vi "机械手.vi"() -> ()   [LabVIEW 2014]
uses:
  <vilib>/Utility/sysdir.llb/System Directory Type.ctl
  <vilib>/Instr/_visa.llb/VISA Configure Serial Port (Instr).vi
panel:
  in  "选项卡控件":enum32{" 肌电传感器电极", " 电机反馈", "FSR&弯曲传感器", "手动写入"}(tab)
  out "手势类型":dbl
  out "蓝牙状态":bool
  in  "接收串口":refnum<visa-resource-name>
  in  "?":bool
  out "肌电传感器电极":dbl(graph)
  out "肌电传感器电极 2":dbl(graph)
  out "肌电传感器电极 3":dbl(graph)
  out "肌电传感器电极 4":dbl(graph)
  out "肌电传感器电极 5":dbl(graph)
  out "肌电传感器电极 6":dbl(graph)
  out "肌电传感器电极 7":dbl(graph)
  out "肌电传感器电极 8":dbl(graph)
  in  "?":bool
  out "小指摆动电机电流":dbl
  out "无名指摆动电机电流":dbl
  out "中指摆动电机电流":dbl
  out "食指摆动电机电流":dbl
  out "拇指摆动电机电流":dbl
  out "拇指张合电机电流":dbl
  out "中指摆动电机转速":dbl(graph)
  out "无名指摆动电机转速":dbl(graph)
  out "小指摆动电机转速":dbl(graph)
  out "拇指张合电机转速":dbl(graph)
  out "拇指摆动电机转速":dbl(graph)
  out "食指摆动电机转速":dbl(graph)
  in  "?":bool
  out "复合":dynamicdata(graph)
  out "FSR4法向压力 4":dbl(graph)
  out "拇指弯曲度":dbl(graph)
  out "食指弯曲度":dbl(graph)
  out "中指弯曲度":dbl(graph)
  out "FSR1法向压力":dbl(graph)
  out "FSR2法向压力":dbl(graph)
  out "FSR3法向压力":dbl(graph)
  out "数值显示控件 6":dbl
  out "数值显示控件 5":dbl
  out "数值显示控件 4":dbl
  out "数值显示控件 3":dbl
  out "数值显示控件 2":dbl
  out "数值显示控件":dbl
  in  "?":bool
  in  "?":bool
  in  "?":bool
  in  "?":bool
  in  "?":bool
  in  "?":bool
  in  "?":bool
  in  "?":bool
  in  "小指摆动电机目标转速":dbl(knob) scale=-29.286..29.286 scale format="%#_4g"
  in  "无名指摆动电机目标转速":dbl(knob) scale=-29.286..29.286 scale format="%#_4g"
  in  "中指摆动电机目标转速":dbl(knob) scale=-29.286..29.286 scale format="%#_4g"
  in  "食指摆动电机目标转速":dbl(knob) scale=-29.286..29.286 scale format="%#_4g"
  in  "拇指摆动电机目标转速":dbl(knob) scale=-29.286..29.286 scale format="%#_4g"
  in  "拇指张合电机目标转速":dbl(knob) scale=-29.286..29.286 scale format="%#_4g"
  # "中南大学机电工程学院 复杂装备智能控制实验室  假肢手控制系统V2.0"
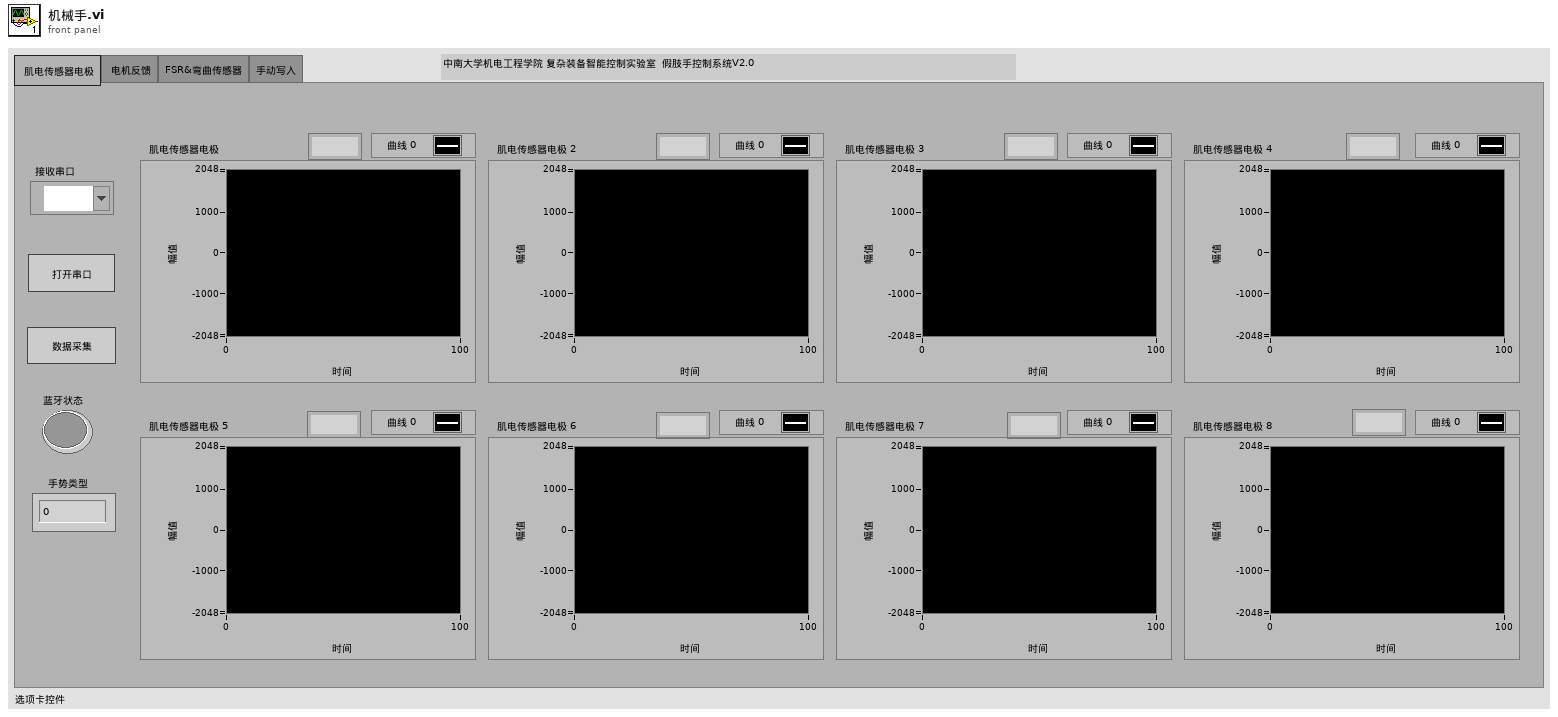
[diagram p1: front panel]
types:
  T1 = enum16{"open", "replace", "create", "open or create", "replace or create", "replace or create with confirmation"}
  T2 = typedef "System Directory Type.ctl" = i32
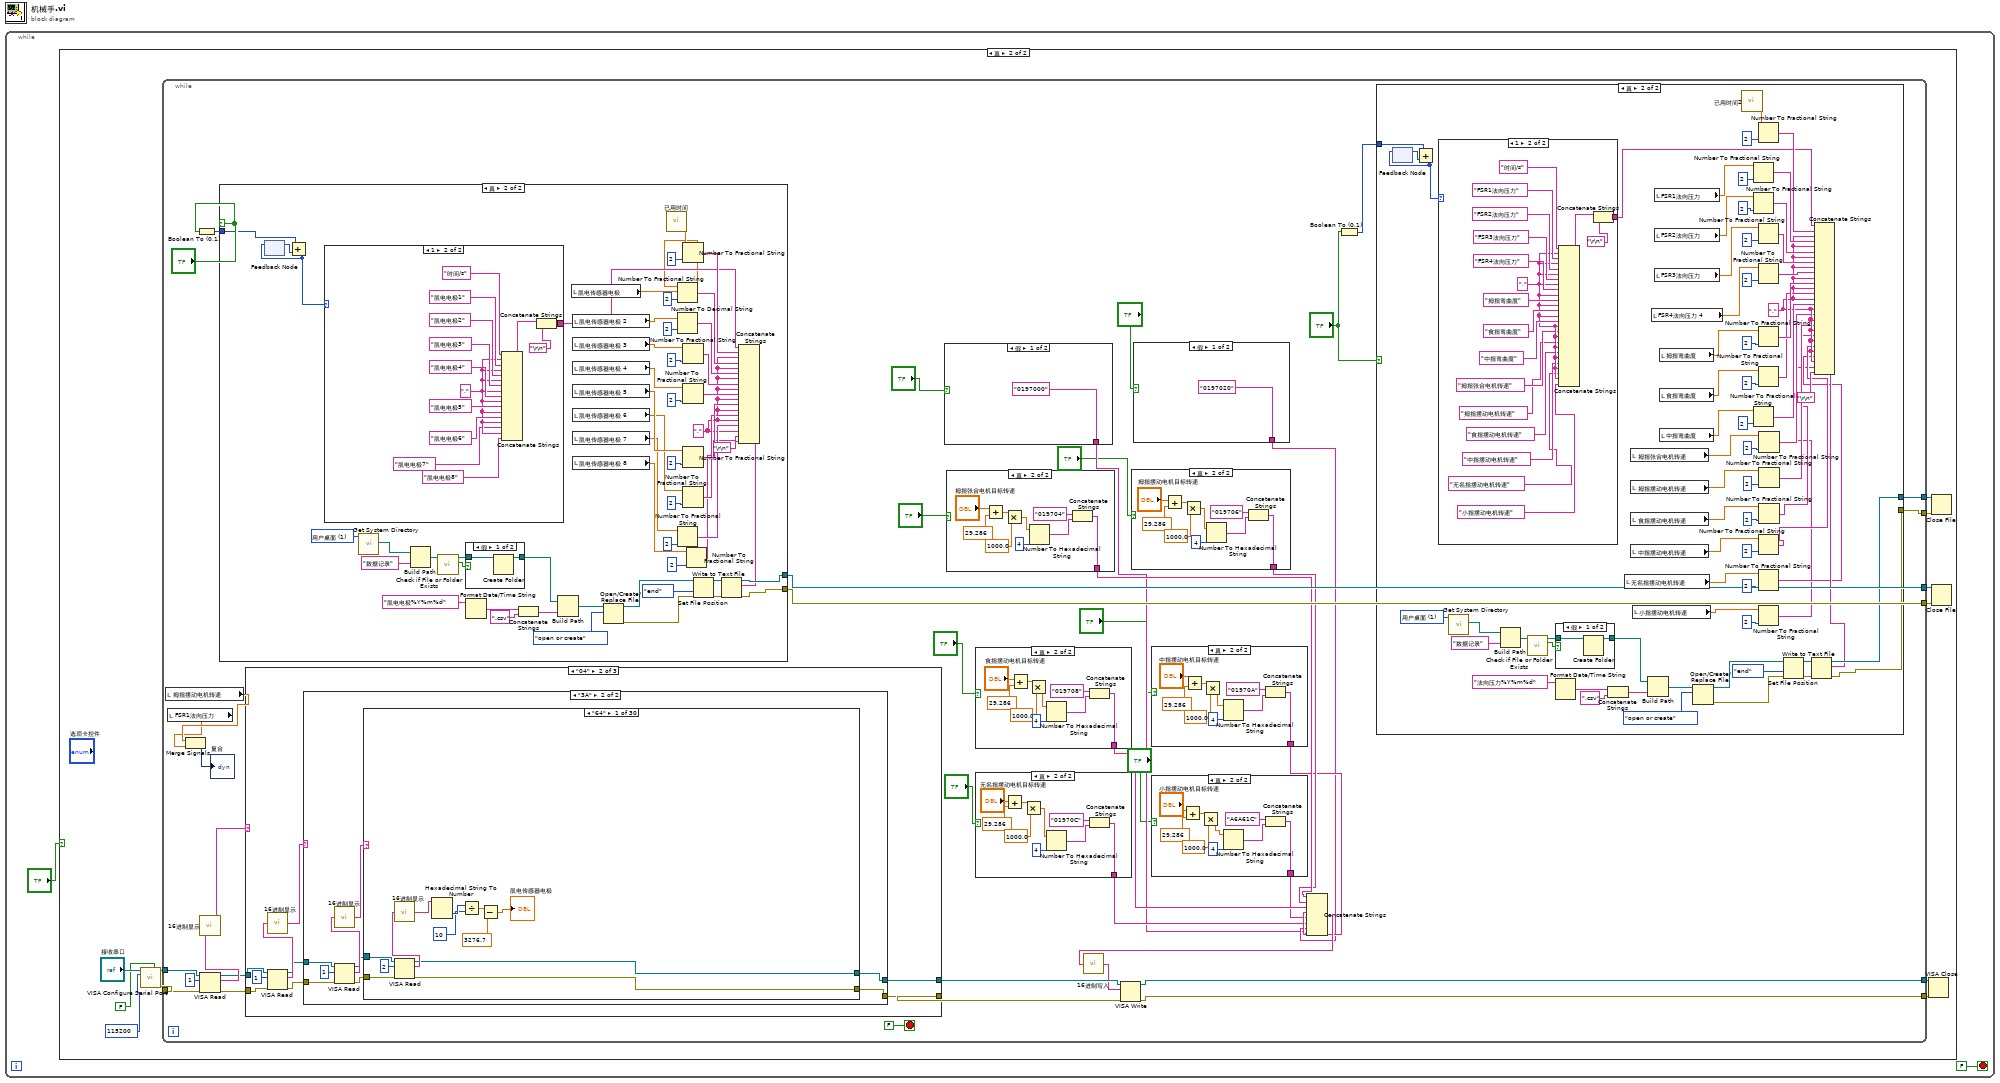
[diagram p0: block diagram]
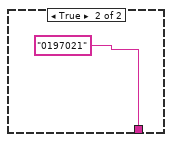
[diagram p6: hidden frame]
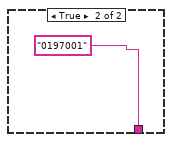
[diagram p7: hidden frame]
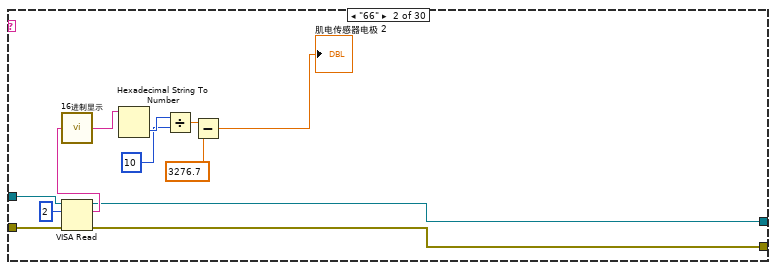
[diagram p19: hidden frame]
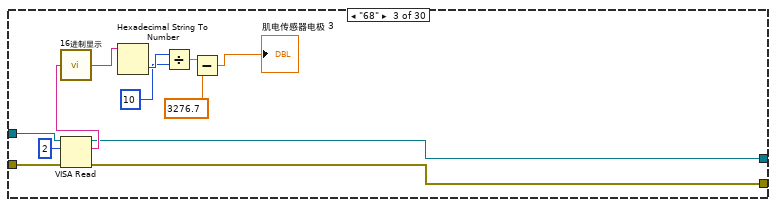
[diagram p20: hidden frame]
diagram:
  n1 = while {
    stop <- FALSE stop-if-true
    n2 = case shown="真" "?" {
      frame False {
      }
      frame True {
        n3 = call-poly "VISA Configure Serial Port"("VISA resource name"="接收串口", "Enable Termination\nChar (T)"=FALSE ("Enable Termination\nChar (T)"), "baud rate (9600)"=u32 115200) -> ("VISA resource name out"=w10:refnum<visa-resource-name>, "error out"=w9:errorcluster)  [unwired: 11 in]
        n4 = while {
          tunnel: w10 -> [w52]
          tunnel: w9 -> [w51]
          tunnel: [w37] -> w8
          tunnel: [w36] -> w7
          tunnel: [w44] -> w6
          tunnel: [w43] -> w5
          tunnel: [w17] -> w4
          tunnel: [w16] -> w3
          stop <- FALSE stop-if-true
          n5 = local read "拇指摆动电机转速"() -> (w41:dbl)
          n6 = local read "FSR1法向压力"() -> (w40:dbl)
          n7 = Merge Signals(w41, w40) -> (→"复合":dynamicdata)
          n8 = Boolean To (0,1)(Boolean="?") -> (0, 1=w46:i16)
          n9 = VISA Read(VISA resource name=w52, byte count=u32 1 ("字节总数"), error in (no error)=w51) -> (VISA resource name out=w48:refnum<visa-resource-name>, read buffer=w50:string, error out=w47:errorcluster)  [unwired: 1 out]
          n10 = call "16进制显示.vi"("输入"=w50) -> ("输出"=w49:string)
          n11 = case shown="真" "?" {
            tunnel: [_ w256] -> w44
            tunnel: [_ w255] -> w43
            tunnel: w46 -> [_ w254]
            frame False {
            }
            frame True {
              w203 = "," ("字符串")
              w231 = T2 1 items=["用户目录"=0, "用户桌面"=1, "用户文档"=2, "用户应用程序数据"=3, "用户设置"=4, "用户临时目录"=5, "公共文档"=6, "公共应用程序数据"=7, "公共设置"=8, "公共缓存"=13, "系统核心库"=9, "系统安装库"=10, "应用程序文件"=11, "启动盘根目录"=12] ("system directory type")
              n12 = feedback #1() -> (w233:i16)  [unwired: 1 in]
              n13 = Add(x=w254, y=w233) -> (x+y=w232:i16)
              n14 = feedback-in #1(w232) -> ()
              n15 = case shown="1" w232 {
                tunnel: [_ w261] -> w219
                frame 0, Default {
                }
                frame 1 {
                  w262 = "," ("字符串")
                  n16 = Concatenate Strings("时间/s" ("字符串"), w262, "肌电电极1" ("字符串"), w262, "肌电电极2" ("字符串"), w262, "肌电电极3" ("字符串"), w262, "肌电电极4" ("字符串"), w262, "肌电电极5" ("字符串"), w262, "肌电电极6" ("字符串"), w262, "肌电电极7" ("字符串"), w262, "肌电电极8" ("字符串")) -> (w260:string)
                  n17 = Concatenate Strings(w260, "\r\n") -> (w261:string)
                }
              }
              n18 = call <vilib>:"Get System Directory.vi"("system directory type"=w231) -> ("system directory"=w230:path)  [unwired: 10 in]
              n19 = Build Path(base path=w230, name or relative path="数据记录" ("名称或相对路径")) -> (appended path=w253:path)
              n20 = call <vilib>:"Check if File or Folder Exists.vi"("path"=w253) -> ("file or folder exists?"=w251:bool, "dup path"=w252:path)  [unwired: 8 in, 1 out]
              n21 = case shown="假" w251 {
                tunnel: w252 -> [w271 w272]
                tunnel: [w270 w272] -> w240
                frame False {
                  n22 = Create Folder(path (use dialog)=w271) -> (created path=w270:path)  [unwired: 2 in, 2 out]
                }
                frame True {
                }
              }
              n23 = Format Date/Time String(time format string (%c)="肌电电极%Y%m%d" ("时间格式字符串(%c)")) -> (date/time string=w239:string)  [unwired: 2 in]
              n24 = Concatenate Strings(w239, ".csv" ("字符串")) -> (w245:string)
              n25 = Build Path(base path=w240, name or relative path=w245) -> (appended path=w247:path)
              n26 = local read "肌电传感器电极"() -> (w217:dbl)
              n27 = local read "肌电传感器电极 2"() -> (w214:dbl)
              n28 = local read "肌电传感器电极 3"() -> (w213:dbl)
              n29 = local read "肌电传感器电极 4"() -> (w212:dbl)
              n30 = local read "肌电传感器电极 5"() -> (w211:dbl)
              n31 = local read "肌电传感器电极 6"() -> (w210:dbl)
              n32 = local read "肌电传感器电极 7"() -> (w209:dbl)
              n33 = local read "肌电传感器电极 8"() -> (w205:dbl)
              n34 = Open/Create/Replace File(file path (use dialog)=w247, operation (0:open)=T1."open or create" ("操作(0:open)")) -> (refnum out=w248:refnum<file>, error out=w249:errorcluster)  [unwired: 4 in, 1 out]
              n35 = call "已用时间"() -> ("Elapsed Time (s)"=w236:dbl)  [unwired: 12 in, 7 out]
              n36 = Number To Fractional String(number=w217, precision (6)=i16 2 ("精度(6)")) -> (F-format string=w221:string)  [unwired: 2 in]
              n37 = Number To Decimal String(number=w214, width (-)=i16 2 ("宽度(-)")) -> (decimal integer string=w208:string)
              n38 = Number To Fractional String(number=w209, precision (6)=i16 2 ("精度(6)")) -> (F-format string=w220:string)  [unwired: 2 in]
              n39 = Number To Fractional String(number=w236, precision (6)=i16 2 ("精度(6)")) -> (F-format string=w235:string)  [unwired: 2 in]
              n40 = Number To Fractional String(number=w213, precision (6)=i16 2 ("精度(6)")) -> (F-format string=w229:string)  [unwired: 2 in]
              n41 = Number To Fractional String(number=w212, precision (6)=i16 2 ("精度(6)")) -> (F-format string=w228:string)  [unwired: 2 in]
              n42 = Number To Fractional String(number=w211, precision (6)=i16 2 ("精度(6)")) -> (F-format string=w227:string)  [unwired: 2 in]
              n43 = Number To Fractional String(number=w210, precision (6)=i16 2 ("精度(6)")) -> (F-format string=w226:string)  [unwired: 2 in]
              n44 = Number To Fractional String(number=w205, precision (6)=i16 2 ("精度(6)")) -> (F-format string=w204:string)  [unwired: 2 in]
              n45 = Set File Position(refnum=w248, from (0:start)=enum16{"start", "end", "current"}."end" ("自（0:起始）"), error in=w249) -> (refnum out=w243:refnum<file>, error out=w242:errorcluster)  [unwired: 1 in]
              n46 = Concatenate Strings(w219, w235, w203, w221, w203, w208, w203, w229, w203, w228, w203, w227, w203, w226, w203, w220, w203, w204, "\r\n") -> (w237:string)
              n47 = Write to Text File(file (use dialog)=w243, text=w237, error in=w242) -> (refnum out=w256:refnum<file>, error out=w255:errorcluster)  [unwired: 1 in, 1 out]
            }
          }
          n48 = case shown="\"04\"" w49 {
            tunnel: w48 -> [w274 w282 w607]
            tunnel: w47 -> [w273 w281 w606]
            tunnel: [w274 w276 w602] -> w39
            tunnel: [w273 w275 w601] -> w38
            frame "假", Default {
            }
            frame "04" {
              n49 = VISA Read(VISA resource name=w282, byte count=u32 1 ("字节总数"), error in (no error)=w281) -> (VISA resource name out=w279:refnum<visa-resource-name>, read buffer=w280:string, error out=w278:errorcluster)  [unwired: 1 out]
              n50 = call "16进制显示.vi"("输入"=w280) -> ("输出"=w277:string)
              n51 = case shown="\"3A\"" w277 {
                tunnel: w279 -> [w285 w293]
                tunnel: w278 -> [w284 w292]
                tunnel: [w285 w287] -> w276
                tunnel: [w284 w286] -> w275
                frame "假", Default {
                }
                frame "3A" {
                  n52 = VISA Read(VISA resource name=w293, byte count=u32 1 ("字节总数"), error in (no error)=w292) -> (VISA resource name out=w289:refnum<visa-resource-name>, read buffer=w291:string, error out=w288:errorcluster)  [unwired: 1 out]
                  n53 = call "16进制显示.vi"("输入"=w291) -> ("输出"=w290:string)
                  n54 = case shown="\"64\"" w290 {
                    tunnel: w289 -> [w305 w311 w323 w335 w347 w359 w371 w383 w395 w407 w419 w431 w443 w455 w467 w475 w483 w491 w499 w507 w517 w527 w537 w547 w557 w567 w577 w585 w595 w600]
                    tunnel: w288 -> [w304 w310 w322 w334 w346 w358 w370 w382 w394 w406 w418 w430 w442 w454 w466 w474 w482 w490 w498 w506 w516 w526 w536 w546 w556 w566 w576 w584 w594 w599]
                    tunnel: [w302 w309 w321 w333 w345 w357 w369 w381 w393 w405 w417 w429 w441 w453 w465 w473 w481 w489 w497 w505 w515 w525 w535 w545 w555 w565 w575 w583 w593 w600] -> w287
                    tunnel: [w301 w308 w320 w332 w344 w356 w368 w380 w392 w404 w416 w428 w440 w452 w464 w472 w480 w488 w496 w504 w514 w524 w534 w544 w554 w564 w574 w582 w589 w599] -> w286
                    frame "64" {
                      n55 = VISA Read(VISA resource name=w305, byte count=u32 2 ("字节总数"), error in (no error)=w304) -> (VISA resource name out=w302:refnum<visa-resource-name>, read buffer=w303:string, error out=w301:errorcluster)  [unwired: 1 out]
                      n56 = call "16进制显示.vi"("输入"=w303) -> ("输出"=w300:string)
                      n57 = Hexadecimal String To Number(string=w300) -> (number=w299:u32)  [unwired: 2 in, 1 out]
                      n58 = Divide(x=w299, y=u32 10) -> (x/y=w297:dbl)
                      n59 = Subtract(x=w297, y=3276.7) -> (x-y=→"肌电传感器电极":dbl)
                    }
                    frame "66" {
                      n60 = VISA Read(VISA resource name=w311, byte count=u32 2 ("字节总数"), error in (no error)=w310) -> (VISA resource name out=w309:refnum<visa-resource-name>, read buffer=w317:string, error out=w308:errorcluster)  [unwired: 1 out]
                      n61 = call "16进制显示.vi"("输入"=w317) -> ("输出"=w316:string)
                      n62 = Hexadecimal String To Number(string=w316) -> (number=w315:u32)  [unwired: 2 in, 1 out]
                      n63 = Divide(x=w315, y=u32 10) -> (x/y=w313:dbl)
                      n64 = Subtract(x=w313, y=3276.7) -> (x-y=→"肌电传感器电极 2":dbl)
                    }
                    frame "68" {
                      n65 = VISA Read(VISA resource name=w323, byte count=u32 2 ("字节总数"), error in (no error)=w322) -> (VISA resource name out=w321:refnum<visa-resource-name>, read buffer=w329:string, error out=w320:errorcluster)  [unwired: 1 out]
                      n66 = call "16进制显示.vi"("输入"=w329) -> ("输出"=w328:string)
                      n67 = Hexadecimal String To Number(string=w328) -> (number=w327:u32)  [unwired: 2 in, 1 out]
                      n68 = Divide(x=w327, y=u32 10) -> (x/y=w325:dbl)
                      n69 = Subtract(x=w325, y=3276.7) -> (x-y=→"肌电传感器电极 3":dbl)
                    }
                    frame "6A" {
                      n70 = VISA Read(VISA resource name=w335, byte count=u32 2 ("字节总数"), error in (no error)=w334) -> (VISA resource name out=w333:refnum<visa-resource-name>, read buffer=w341:string, error out=w332:errorcluster)  [unwired: 1 out]
                      n71 = call "16进制显示.vi"("输入"=w341) -> ("输出"=w340:string)
                      n72 = Hexadecimal String To Number(string=w340) -> (number=w339:u32)  [unwired: 2 in, 1 out]
                      n73 = Divide(x=w339, y=u32 10) -> (x/y=w337:dbl)
                      n74 = Subtract(x=w337, y=3276.7) -> (x-y=→"肌电传感器电极 4":dbl)
                    }
                    frame "6C" {
                      n75 = VISA Read(VISA resource name=w347, byte count=u32 2 ("字节总数"), error in (no error)=w346) -> (VISA resource name out=w345:refnum<visa-resource-name>, read buffer=w353:string, error out=w344:errorcluster)  [unwired: 1 out]
                      n76 = call "16进制显示.vi"("输入"=w353) -> ("输出"=w352:string)
                      n77 = Hexadecimal String To Number(string=w352) -> (number=w351:u32)  [unwired: 2 in, 1 out]
                      n78 = Divide(x=w351, y=u32 10) -> (x/y=w349:dbl)
                      n79 = Subtract(x=w349, y=3276.7) -> (x-y=→"肌电传感器电极 5":dbl)
                    }
                    frame "6E" {
                      n80 = VISA Read(VISA resource name=w359, byte count=u32 2 ("字节总数"), error in (no error)=w358) -> (VISA resource name out=w357:refnum<visa-resource-name>, read buffer=w365:string, error out=w356:errorcluster)  [unwired: 1 out]
                      n81 = call "16进制显示.vi"("输入"=w365) -> ("输出"=w364:string)
                      n82 = Hexadecimal String To Number(string=w364) -> (number=w363:u32)  [unwired: 2 in, 1 out]
                      n83 = Divide(x=w363, y=u32 10) -> (x/y=w361:dbl)
                      n84 = Subtract(x=w361, y=3276.7) -> (x-y=→"肌电传感器电极 6":dbl)
                    }
                    frame "70" {
                      n85 = VISA Read(VISA resource name=w371, byte count=u32 2 ("字节总数"), error in (no error)=w370) -> (VISA resource name out=w369:refnum<visa-resource-name>, read buffer=w377:string, error out=w368:errorcluster)  [unwired: 1 out]
                      n86 = call "16进制显示.vi"("输入"=w377) -> ("输出"=w376:string)
                      n87 = Hexadecimal String To Number(string=w376) -> (number=w375:u32)  [unwired: 2 in, 1 out]
                      n88 = Divide(x=w375, y=u32 10) -> (x/y=w373:dbl)
                      n89 = Subtract(x=w373, y=3276.7) -> (x-y=→"肌电传感器电极 7":dbl)
                    }
                    frame "72" {
                      n90 = VISA Read(VISA resource name=w383, byte count=u32 2 ("字节总数"), error in (no error)=w382) -> (VISA resource name out=w381:refnum<visa-resource-name>, read buffer=w389:string, error out=w380:errorcluster)  [unwired: 1 out]
                      n91 = call "16进制显示.vi"("输入"=w389) -> ("输出"=w388:string)
                      n92 = Hexadecimal String To Number(string=w388) -> (number=w387:u32)  [unwired: 2 in, 1 out]
                      n93 = Divide(x=w387, y=u32 10) -> (x/y=w385:dbl)
                      n94 = Subtract(x=w385, y=3276.7) -> (x-y=→"肌电传感器电极 8":dbl)
                    }
                    frame "74" {
                      n95 = VISA Read(VISA resource name=w395, byte count=u32 2 ("字节总数"), error in (no error)=w394) -> (VISA resource name out=w393:refnum<visa-resource-name>, read buffer=w401:string, error out=w392:errorcluster)  [unwired: 1 out]
                      n96 = call "16进制显示.vi"("输入"=w401) -> ("输出"=w400:string)
                      n97 = Hexadecimal String To Number(string=w400) -> (number=w399:u32)  [unwired: 2 in, 1 out]
                      n98 = Divide(x=w399, y=u32 1000) -> (x/y=w397:dbl)
                      n99 = Subtract(x=w397, y=29.286) -> (x-y=→"拇指张合电机转速":dbl)
                    }
                    frame "76" {
                      n100 = VISA Read(VISA resource name=w407, byte count=u32 2 ("字节总数"), error in (no error)=w406) -> (VISA resource name out=w405:refnum<visa-resource-name>, read buffer=w413:string, error out=w404:errorcluster)  [unwired: 1 out]
                      n101 = call "16进制显示.vi"("输入"=w413) -> ("输出"=w412:string)
                      n102 = Hexadecimal String To Number(string=w412) -> (number=w411:u32)  [unwired: 2 in, 1 out]
                      n103 = Divide(x=w411, y=u32 1000) -> (x/y=w409:dbl)
                      n104 = Subtract(x=w409, y=29.286) -> (x-y=→"拇指摆动电机转速":dbl)
                    }
                    frame "78" {
                      n105 = VISA Read(VISA resource name=w419, byte count=u32 2 ("字节总数"), error in (no error)=w418) -> (VISA resource name out=w417:refnum<visa-resource-name>, read buffer=w425:string, error out=w416:errorcluster)  [unwired: 1 out]
                      n106 = call "16进制显示.vi"("输入"=w425) -> ("输出"=w424:string)
                      n107 = Hexadecimal String To Number(string=w424) -> (number=w423:u32)  [unwired: 2 in, 1 out]
                      n108 = Divide(x=w423, y=u32 1000) -> (x/y=w421:dbl)
                      n109 = Subtract(x=w421, y=29.286) -> (x-y=→"食指摆动电机转速":dbl)
                    }
                    frame "7A" {
                      n110 = VISA Read(VISA resource name=w431, byte count=u32 2 ("字节总数"), error in (no error)=w430) -> (VISA resource name out=w429:refnum<visa-resource-name>, read buffer=w437:string, error out=w428:errorcluster)  [unwired: 1 out]
                      n111 = call "16进制显示.vi"("输入"=w437) -> ("输出"=w436:string)
                      n112 = Hexadecimal String To Number(string=w436) -> (number=w435:u32)  [unwired: 2 in, 1 out]
                      n113 = Divide(x=w435, y=u32 1000) -> (x/y=w433:dbl)
                      n114 = Subtract(x=w433, y=29.286) -> (x-y=→"中指摆动电机转速":dbl)
                    }
                    frame "7C" {
                      n115 = VISA Read(VISA resource name=w443, byte count=u32 2 ("字节总数"), error in (no error)=w442) -> (VISA resource name out=w441:refnum<visa-resource-name>, read buffer=w449:string, error out=w440:errorcluster)  [unwired: 1 out]
                      n116 = call "16进制显示.vi"("输入"=w449) -> ("输出"=w448:string)
                      n117 = Hexadecimal String To Number(string=w448) -> (number=w447:u32)  [unwired: 2 in, 1 out]
                      n118 = Divide(x=w447, y=u32 1000) -> (x/y=w445:dbl)
                      n119 = Subtract(x=w445, y=29.286) -> (x-y=→"无名指摆动电机转速":dbl)
                    }
                    frame "7E" {
                      n120 = VISA Read(VISA resource name=w455, byte count=u32 2 ("字节总数"), error in (no error)=w454) -> (VISA resource name out=w453:refnum<visa-resource-name>, read buffer=w461:string, error out=w452:errorcluster)  [unwired: 1 out]
                      n121 = call "16进制显示.vi"("输入"=w461) -> ("输出"=w460:string)
                      n122 = Hexadecimal String To Number(string=w460) -> (number=w459:u32)  [unwired: 2 in, 1 out]
                      n123 = Divide(x=w459, y=u32 1000) -> (x/y=w457:dbl)
                      n124 = Subtract(x=w457, y=29.286) -> (x-y=→"小指摆动电机转速":dbl)
                    }
                    frame "80" {
                      n125 = VISA Read(VISA resource name=w467, byte count=u32 2 ("字节总数"), error in (no error)=w466) -> (VISA resource name out=w465:refnum<visa-resource-name>, read buffer=w469:string, error out=w464:errorcluster)  [unwired: 1 out]
                      n126 = call "16进制显示.vi"("输入"=w469) -> ("输出"=w468:string)
                      n127 = Hexadecimal String To Number(string=w468) -> (number=→"拇指张合电机电流":u32)  [unwired: 2 in, 1 out]
                    }
                    frame "82" {
                      n128 = VISA Read(VISA resource name=w475, byte count=u32 2 ("字节总数"), error in (no error)=w474) -> (VISA resource name out=w473:refnum<visa-resource-name>, read buffer=w477:string, error out=w472:errorcluster)  [unwired: 1 out]
                      n129 = call "16进制显示.vi"("输入"=w477) -> ("输出"=w476:string)
                      n130 = Hexadecimal String To Number(string=w476) -> (number=→"拇指摆动电机电流":u32)  [unwired: 2 in, 1 out]
                    }
                    frame "84" {
                      n131 = VISA Read(VISA resource name=w483, byte count=u32 2 ("字节总数"), error in (no error)=w482) -> (VISA resource name out=w481:refnum<visa-resource-name>, read buffer=w485:string, error out=w480:errorcluster)  [unwired: 1 out]
                      n132 = call "16进制显示.vi"("输入"=w485) -> ("输出"=w484:string)
                      n133 = Hexadecimal String To Number(string=w484) -> (number=→"食指摆动电机电流":u32)  [unwired: 2 in, 1 out]
                    }
                    frame "86" {
                      n134 = VISA Read(VISA resource name=w491, byte count=u32 2 ("字节总数"), error in (no error)=w490) -> (VISA resource name out=w489:refnum<visa-resource-name>, read buffer=w493:string, error out=w488:errorcluster)  [unwired: 1 out]
                      n135 = call "16进制显示.vi"("输入"=w493) -> ("输出"=w492:string)
                      n136 = Hexadecimal String To Number(string=w492) -> (number=→"中指摆动电机电流":u32)  [unwired: 2 in, 1 out]
                    }
                    frame "88" {
                      n137 = VISA Read(VISA resource name=w499, byte count=u32 2 ("字节总数"), error in (no error)=w498) -> (VISA resource name out=w497:refnum<visa-resource-name>, read buffer=w501:string, error out=w496:errorcluster)  [unwired: 1 out]
                      n138 = call "16进制显示.vi"("输入"=w501) -> ("输出"=w500:string)
                      n139 = Hexadecimal String To Number(string=w500) -> (number=→"无名指摆动电机电流":u32)  [unwired: 2 in, 1 out]
                    }
                    frame "8A" {
                      n140 = VISA Read(VISA resource name=w507, byte count=u32 2 ("字节总数"), error in (no error)=w506) -> (VISA resource name out=w505:refnum<visa-resource-name>, read buffer=w509:string, error out=w504:errorcluster)  [unwired: 1 out]
                      n141 = call "16进制显示.vi"("输入"=w509) -> ("输出"=w508:string)
                      n142 = Hexadecimal String To Number(string=w508) -> (number=→"小指摆动电机电流":u32)  [unwired: 2 in, 1 out]
                    }
                    frame "8C" {
                      n143 = VISA Read(VISA resource name=w517, byte count=u32 2 ("字节总数"), error in (no error)=w516) -> (VISA resource name out=w515:refnum<visa-resource-name>, read buffer=w519:string, error out=w514:errorcluster)  [unwired: 1 out]
                      n144 = call "16进制显示.vi"("输入"=w519) -> ("输出"=w518:string)
                      n145 = Hexadecimal String To Number(string=w518) -> (number=w512:u32)  [unwired: 2 in, 1 out]
                      n146 = Divide(x=w512, y=u32 100) -> (x/y=→"FSR1法向压力":dbl)
                    }
                    frame "8E" {
                      n147 = VISA Read(VISA resource name=w527, byte count=u32 2 ("字节总数"), error in (no error)=w526) -> (VISA resource name out=w525:refnum<visa-resource-name>, read buffer=w529:string, error out=w524:errorcluster)  [unwired: 1 out]
                      n148 = call "16进制显示.vi"("输入"=w529) -> ("输出"=w528:string)
                      n149 = Hexadecimal String To Number(string=w528) -> (number=w522:u32)  [unwired: 2 in, 1 out]
                      n150 = Divide(x=w522, y=u32 100) -> (x/y=→"FSR2法向压力":dbl)
                    }
                    frame "90" {
                      n151 = VISA Read(VISA resource name=w537, byte count=u32 2 ("字节总数"), error in (no error)=w536) -> (VISA resource name out=w535:refnum<visa-resource-name>, read buffer=w539:string, error out=w534:errorcluster)  [unwired: 1 out]
                      n152 = call "16进制显示.vi"("输入"=w539) -> ("输出"=w538:string)
                      n153 = Hexadecimal String To Number(string=w538) -> (number=w532:u32)  [unwired: 2 in, 1 out]
                      n154 = Divide(x=w532, y=u32 100) -> (x/y=→"FSR3法向压力":dbl)
                    }
                    frame "92" {
                      n155 = VISA Read(VISA resource name=w547, byte count=u32 2 ("字节总数"), error in (no error)=w546) -> (VISA resource name out=w545:refnum<visa-resource-name>, read buffer=w549:string, error out=w544:errorcluster)  [unwired: 1 out]
                      n156 = call "16进制显示.vi"("输入"=w549) -> ("输出"=w548:string)
                      n157 = Hexadecimal String To Number(string=w548) -> (number=w543:u32)  [unwired: 2 in, 1 out]
                      n158 = Divide(x=w543, y=u32 100) -> (x/y=→"FSR4法向压力 4":dbl)
                    }
                    frame "94" {
                      n159 = VISA Read(VISA resource name=w557, byte count=u32 2 ("字节总数"), error in (no error)=w556) -> (VISA resource name out=w555:refnum<visa-resource-name>, read buffer=w559:string, error out=w554:errorcluster)  [unwired: 1 out]
                      n160 = call "16进制显示.vi"("输入"=w559) -> ("输出"=w558:string)
                      n161 = Hexadecimal String To Number(string=w558) -> (number=w553:u32)  [unwired: 2 in, 1 out]
                      n162 = Divide(x=w553, y=u32 100) -> (x/y=→"拇指弯曲度":dbl)
                    }
                    frame "96" {
                      n163 = VISA Read(VISA resource name=w567, byte count=u32 2 ("字节总数"), error in (no error)=w566) -> (VISA resource name out=w565:refnum<visa-resource-name>, read buffer=w569:string, error out=w564:errorcluster)  [unwired: 1 out]
                      n164 = call "16进制显示.vi"("输入"=w569) -> ("输出"=w568:string)
                      n165 = Hexadecimal String To Number(string=w568) -> (number=w561:u32)  [unwired: 2 in, 1 out]
                      n166 = Divide(x=w561, y=u32 100) -> (x/y=→"食指弯曲度":dbl)
                    }
                    frame "98" {
                      n167 = VISA Read(VISA resource name=w577, byte count=u32 2 ("字节总数"), error in (no error)=w576) -> (VISA resource name out=w575:refnum<visa-resource-name>, read buffer=w579:string, error out=w574:errorcluster)  [unwired: 1 out]
                      n168 = call "16进制显示.vi"("输入"=w579) -> ("输出"=w578:string)
                      n169 = Hexadecimal String To Number(string=w578) -> (number=w572:u32)  [unwired: 2 in, 1 out]
                      n170 = Divide(x=w572, y=u32 100) -> (x/y=→"中指弯曲度":dbl)
                    }
                    frame "9A" {
                      n171 = VISA Read(VISA resource name=w585, byte count=u32 2 ("字节总数"), error in (no error)=w584) -> (VISA resource name out=w583:refnum<visa-resource-name>, read buffer=w587:string, error out=w582:errorcluster)  [unwired: 1 out]
                      n172 = call "16进制显示.vi"("输入"=w587) -> ("输出"=w586:string)
                      n173 = Hexadecimal String To Number(string=w586) -> (number=→"手势类型":u32)  [unwired: 2 in, 1 out]
                    }
                    frame "9C" {
                      n174 = VISA Read(VISA resource name=w595, byte count=u32 2 ("字节总数"), error in (no error)=w594) -> (VISA resource name out=w593:refnum<visa-resource-name>, read buffer=w597:string, error out=w589:errorcluster)  [unwired: 1 out]
                      n175 = call "16进制显示.vi"("输入"=w597) -> ("输出"=w596:string)
                      n176 = Hexadecimal String To Number(string=w596) -> (number=w592:u32)  [unwired: 2 in, 1 out]
                      n177 = Equal?(x=w592, y=u32 1) -> (x = y?=→"蓝牙状态":bool)
                    }
                    frame "假", Default {
                    }
                  }
                }
              }
            }
            frame "01" {
              n178 = VISA Read(VISA resource name=w607, byte count=u32 1 ("字节总数"), error in (no error)=w606) -> (VISA resource name out=w605:refnum<visa-resource-name>, read buffer=w608:string, error out=w604:errorcluster)  [unwired: 1 out]
              n179 = call "16进制显示.vi"("输入"=w608) -> ("输出"=w603:string)
              n180 = case shown="\"97\"" w603 {
                tunnel: w605 -> [w611 w618]
                tunnel: w604 -> [w610 w617]
                tunnel: [w611 w613] -> w602
                tunnel: [w610 w612] -> w601
                frame "假", Default {
                }
                frame "97" {
                  n181 = VISA Read(VISA resource name=w618, byte count=u32 1 ("字节总数"), error in (no error)=w617) -> (VISA resource name out=w616:refnum<visa-resource-name>, read buffer=w619:string, error out=w615:errorcluster)  [unwired: 1 out]
                  n182 = call "16进制显示.vi"("输入"=w619) -> ("输出"=w614:string)
                  n183 = case shown="\"0E\"" w614 {
                    tunnel: w616 -> [w622 w627 w639 w651 w663 w675 w687]
                    tunnel: w615 -> [w621 w626 w638 w650 w662 w674 w686]
                    tunnel: [w622 w625 w637 w649 w661 w673 w685] -> w613
                    tunnel: [w621 w624 w636 w648 w660 w672 w684] -> w612
                    frame "假", Default {
                    }
                    frame "04" {
                      n184 = VISA Read(VISA resource name=w627, byte count=u32 2 ("字节总数"), error in (no error)=w626) -> (VISA resource name out=w625:refnum<visa-resource-name>, read buffer=w633:string, error out=w624:errorcluster)  [unwired: 1 out]
                      n185 = call "16进制显示.vi"("输入"=w633) -> ("输出"=w632:string)
                      n186 = Hexadecimal String To Number(string=w632) -> (number=w631:u32)  [unwired: 2 in, 1 out]
                      n187 = Divide(x=w631, y=u32 1000) -> (x/y=w629:dbl)
                      n188 = Subtract(x=w629, y=29.286) -> (x-y=→"数值显示控件":dbl)
                    }
                    frame "06" {
                      n189 = VISA Read(VISA resource name=w639, byte count=u32 2 ("字节总数"), error in (no error)=w638) -> (VISA resource name out=w637:refnum<visa-resource-name>, read buffer=w645:string, error out=w636:errorcluster)  [unwired: 1 out]
                      n190 = call "16进制显示.vi"("输入"=w645) -> ("输出"=w644:string)
                      n191 = Hexadecimal String To Number(string=w644) -> (number=w643:u32)  [unwired: 2 in, 1 out]
                      n192 = Divide(x=w643, y=u32 1000) -> (x/y=w641:dbl)
                      n193 = Subtract(x=w641, y=29.286) -> (x-y=→"数值显示控件 2":dbl)
                    }
                    frame "08" {
                      n194 = VISA Read(VISA resource name=w651, byte count=u32 2 ("字节总数"), error in (no error)=w650) -> (VISA resource name out=w649:refnum<visa-resource-name>, read buffer=w657:string, error out=w648:errorcluster)  [unwired: 1 out]
                      n195 = call "16进制显示.vi"("输入"=w657) -> ("输出"=w656:string)
                      n196 = Hexadecimal String To Number(string=w656) -> (number=w655:u32)  [unwired: 2 in, 1 out]
                      n197 = Divide(x=w655, y=u32 1000) -> (x/y=w653:dbl)
                      n198 = Subtract(x=w653, y=29.286) -> (x-y=→"数值显示控件 3":dbl)
                    }
                    frame "0A" {
                      n199 = VISA Read(VISA resource name=w663, byte count=u32 2 ("字节总数"), error in (no error)=w662) -> (VISA resource name out=w661:refnum<visa-resource-name>, read buffer=w669:string, error out=w660:errorcluster)  [unwired: 1 out]
                      n200 = call "16进制显示.vi"("输入"=w669) -> ("输出"=w668:string)
                      n201 = Hexadecimal String To Number(string=w668) -> (number=w667:u32)  [unwired: 2 in, 1 out]
                      n202 = Divide(x=w667, y=u32 1000) -> (x/y=w665:dbl)
                      n203 = Subtract(x=w665, y=29.286) -> (x-y=→"数值显示控件 4":dbl)
                    }
                    frame "0C" {
                      n204 = VISA Read(VISA resource name=w675, byte count=u32 2 ("字节总数"), error in (no error)=w674) -> (VISA resource name out=w673:refnum<visa-resource-name>, read buffer=w681:string, error out=w672:errorcluster)  [unwired: 1 out]
                      n205 = call "16进制显示.vi"("输入"=w681) -> ("输出"=w680:string)
                      n206 = Hexadecimal String To Number(string=w680) -> (number=w679:u32)  [unwired: 2 in, 1 out]
                      n207 = Divide(x=w679, y=u32 1000) -> (x/y=w677:dbl)
                      n208 = Subtract(x=w677, y=29.286) -> (x-y=→"数值显示控件 5":dbl)
                    }
                    frame "0E" {
                      n209 = VISA Read(VISA resource name=w687, byte count=u32 2 ("字节总数"), error in (no error)=w686) -> (VISA resource name out=w685:refnum<visa-resource-name>, read buffer=w693:string, error out=w684:errorcluster)  [unwired: 1 out]
                      n210 = call "16进制显示.vi"("输入"=w693) -> ("输出"=w692:string)
                      n211 = Hexadecimal String To Number(string=w692) -> (number=w691:u32)  [unwired: 2 in, 1 out]
                      n212 = Divide(x=w691, y=u32 1000) -> (x/y=w689:dbl)
                      n213 = Subtract(x=w689, y=29.286) -> (x-y=→"数值显示控件 6":dbl)
                    }
                  }
                }
              }
            }
          }
          n214 = case shown="假" "?" {
            tunnel: ["0197000" ("字符串") "0197001" ("字符串")] -> w24
            frame False {
            }
            frame True {
            }
          }
          n215 = case shown="真" "?" {
            tunnel: [_ w199] -> w33
            frame False {
            }
            frame True {
              n216 = Add(x="拇指张合电机目标转速", y=29.286) -> (x+y=w197:dbl)
              n217 = Multiply(x=w197, y=1000.0) -> (x*y=w195:dbl)
              n218 = Number To Hexadecimal String(1:i16 4 ("宽度(-)"), 2:w195) -> (0:w201:string)
              n219 = Concatenate Strings("019704" ("字符串"), w201) -> (w199:string)
            }
          }
          n220 = case shown="真" "?" {
            tunnel: [_ w181] -> w31
            frame False {
            }
            frame True {
              n221 = Add(x="食指摆动电机目标转速", y=29.286) -> (x+y=w179:dbl)
              n222 = Multiply(x=w179, y=1000.0) -> (x*y=w177:dbl)
              n223 = Number To Hexadecimal String(1:i16 4 ("宽度(-)"), 2:w177) -> (0:w183:string)
              n224 = Concatenate Strings("019708" ("字符串"), w183) -> (w181:string)
            }
          }
          n225 = case shown="真" "?" {
            tunnel: [_ w163] -> w28
            frame False {
            }
            frame True {
              n226 = Add(x="无名指摆动电机目标转速", y=29.286) -> (x+y=w161:dbl)
              n227 = Multiply(x=w161, y=1000.0) -> (x*y=w159:dbl)
              n228 = Number To Hexadecimal String(1:i16 4 ("宽度(-)"), 2:w159) -> (0:w165:string)
              n229 = Concatenate Strings("01970C" ("字符串"), w165) -> (w163:string)
            }
          }
          n230 = case shown="真" "?" {
            tunnel: [_ w190] -> w32
            frame False {
            }
            frame True {
              n231 = Add(x="拇指摆动电机目标转速", y=29.286) -> (x+y=w188:dbl)
              n232 = Multiply(x=w188, y=1000.0) -> (x*y=w186:dbl)
              n233 = Number To Hexadecimal String(1:i16 4 ("宽度(-)"), 2:w186) -> (0:w192:string)
              n234 = Concatenate Strings("019706" ("字符串"), w192) -> (w190:string)
            }
          }
          n235 = case shown="假" "?" {
            tunnel: ["0197020" ("字符串") "0197021" ("字符串")] -> w25
            frame False {
            }
            frame True {
            }
          }
          n236 = case shown="真" "?" {
            tunnel: [_ w172] -> w30
            frame False {
            }
            frame True {
              n237 = Add(x="中指摆动电机目标转速", y=29.286) -> (x+y=w170:dbl)
              n238 = Multiply(x=w170, y=1000.0) -> (x*y=w168:dbl)
              n239 = Number To Hexadecimal String(1:i16 4 ("宽度(-)"), 2:w168) -> (0:w174:string)
              n240 = Concatenate Strings("01970A" ("字符串"), w174) -> (w172:string)
            }
          }
          n241 = case shown="真" "?" {
            tunnel: [_ w154] -> w29
            frame False {
            }
            frame True {
              n242 = Add(x="小指摆动电机目标转速", y=29.286) -> (x+y=w152:dbl)
              n243 = Multiply(x=w152, y=1000.0) -> (x*y=w150:dbl)
              n244 = Number To Hexadecimal String(1:i16 4 ("宽度(-)"), 2:w150) -> (0:w156:string)
              n245 = Concatenate Strings("A6A61C" ("字符串"), w156) -> (w154:string)
            }
          }
          n246 = Concatenate Strings(w33, w32, w31, w30, w29, w28, w25, w24) -> (w34:string)
          n247 = call "16进制写入.vi"("输入"=w34) -> ("输出"=w35:string)
          n248 = VISA Write(VISA resource name=w39, write buffer=w35, error in (no error)=w38) -> (VISA resource name out=w37:refnum<visa-resource-name>, error out=w36:errorcluster)  [unwired: 1 out]
          n249 = Boolean To (0,1)(Boolean="?") -> (0, 1=w14:i16)
          n250 = case shown="真" "?" {
            tunnel: [_ w105] -> w17
            tunnel: [_ w104] -> w16
            tunnel: w14 -> [_ w101]
            frame False {
            }
            frame True {
              w74 = "," ("字符串")
              w107 = T2 1 items=["用户目录"=0, "用户桌面"=1, "用户文档"=2, "用户应用程序数据"=3, "用户设置"=4, "用户临时目录"=5, "公共文档"=6, "公共应用程序数据"=7, "公共设置"=8, "公共缓存"=13, "系统核心库"=9, "系统安装库"=10, "应用程序文件"=11, "启动盘根目录"=12] ("system directory type")
              n251 = feedback #2() -> (w103:i16)  [unwired: 1 in]
              n252 = Add(x=w101, y=w103) -> (x+y=w102:i16)
              n253 = feedback-in #2(w102) -> ()
              n254 = case shown="1" w102 {
                tunnel: [_ w134] -> w82
                frame 0, Default {
                }
                frame 1 {
                  w130 = "," ("字符串")
                  n255 = Concatenate Strings("时间/s" ("字符串"), w130, "FSR1法向压力" ("字符串"), w130, "FSR2法向压力" ("字符串"), w130, "FSR3法向压力" ("字符串"), w130, "FSR4法向压力" ("字符串"), w130, "拇指弯曲度" ("字符串"), w130, "食指弯曲度" ("字符串"), w130, "中指弯曲度" ("字符串"), w130, "拇指张合电机转速" ("字符串"), w130, "拇指摆动电机转速" ("字符串"), w130, "食指摆动电机转速" ("字符串"), w130, "中指摆动电机转速" ("字符串"), w130, "无名指摆动电机转速" ("字符串"), w130, "小指摆动电机转速" ("字符串")) -> (w133:string)
                  n256 = Concatenate Strings(w133, "\r\n") -> (w134:string)
                }
              }
              n257 = call <vilib>:"Get System Directory.vi"("system directory type"=w107) -> ("system directory"=w106:path)  [unwired: 10 in]
              n258 = Build Path(base path=w106, name or relative path="数据记录" ("名称或相对路径")) -> (appended path=w123:path)
              n259 = call <vilib>:"Check if File or Folder Exists.vi"("path"=w123) -> ("file or folder exists?"=w121:bool, "dup path"=w122:path)  [unwired: 8 in, 1 out]
              n260 = case shown="假" w121 {
                tunnel: w122 -> [w143 w144]
                tunnel: [w142 w144] -> w110
                frame False {
                  n261 = Create Folder(path (use dialog)=w143) -> (created path=w142:path)  [unwired: 2 in, 2 out]
                }
                frame True {
                }
              }
              n262 = Format Date/Time String(time format string (%c)="法向压力%Y%m%d" ("时间格式字符串(%c)")) -> (date/time string=w109:string)  [unwired: 2 in]
              n263 = Concatenate Strings(w109, ".csv" ("字符串")) -> (w115:string)
              n264 = local read "无名指摆动电机转速"() -> (w55:dbl)
              n265 = local read "拇指张合电机转速"() -> (w60:dbl)
              n266 = local read "拇指摆动电机转速"() -> (w59:dbl)
              n267 = local read "食指摆动电机转速"() -> (w58:dbl)
              n268 = local read "中指摆动电机转速"() -> (w57:dbl)
              n269 = local read "小指摆动电机转速"() -> (w56:dbl)
              n270 = Build Path(base path=w110, name or relative path=w115) -> (appended path=w117:path)
              n271 = local read "FSR4法向压力 4"() -> (w78:dbl)
              n272 = local read "FSR1法向压力"() -> (w81:dbl)
              n273 = local read "FSR2法向压力"() -> (w80:dbl)
              n274 = local read "FSR3法向压力"() -> (w79:dbl)
              n275 = local read "拇指弯曲度"() -> (w77:dbl)
              n276 = local read "食指弯曲度"() -> (w76:dbl)
              n277 = local read "中指弯曲度"() -> (w75:dbl)
              n278 = Open/Create/Replace File(file path (use dialog)=w117, operation (0:open)=T1."open or create" ("操作(0:open)")) -> (refnum out=w118:refnum<file>, error out=w119:errorcluster)  [unwired: 4 in, 1 out]
              n279 = call "已用时间2"() -> ("Elapsed Time (s)"=w100:dbl)  [unwired: 12 in, 7 out]
              n280 = Number To Fractional String(number=w81, precision (6)=i16 2 ("精度(6)")) -> (F-format string=w89:string)  [unwired: 2 in]
              n281 = Number To Fractional String(number=w80, precision (6)=i16 2 ("宽度(-)")) -> (F-format string=w85:string)  [unwired: 2 in]
              n282 = Number To Fractional String(number=w75, precision (6)=i16 2 ("精度(6)")) -> (F-format string=w88:string)  [unwired: 2 in]
              n283 = Number To Fractional String(number=w100, precision (6)=i16 2 ("精度(6)")) -> (F-format string=w99:string)  [unwired: 2 in]
              n284 = Number To Fractional String(number=w79, precision (6)=i16 2 ("精度(6)")) -> (F-format string=w97:string)  [unwired: 2 in]
              n285 = Number To Fractional String(number=w78, precision (6)=i16 2 ("精度(6)")) -> (F-format string=w96:string)  [unwired: 2 in]
              n286 = Number To Fractional String(number=w77, precision (6)=i16 2 ("精度(6)")) -> (F-format string=w95:string)  [unwired: 2 in]
              n287 = Number To Fractional String(number=w76, precision (6)=i16 2 ("精度(6)")) -> (F-format string=w94:string)  [unwired: 2 in]
              n288 = Number To Fractional String(number=w57, precision (6)=i16 2 ("精度(6)")) -> (F-format string=w63:string)  [unwired: 2 in]
              n289 = Number To Fractional String(number=w55, precision (6)=i16 2 ("精度(6)")) -> (F-format string=w62:string)  [unwired: 2 in]
              n290 = Number To Fractional String(number=w56, precision (6)=i16 2 ("精度(6)")) -> (F-format string=w61:string)  [unwired: 2 in]
              n291 = Number To Fractional String(number=w60, precision (6)=i16 2 ("精度(6)")) -> (F-format string=w66:string)  [unwired: 2 in]
              n292 = Number To Fractional String(number=w59, precision (6)=i16 2 ("精度(6)")) -> (F-format string=w65:string)  [unwired: 2 in]
              n293 = Number To Fractional String(number=w58, precision (6)=i16 2 ("精度(6)")) -> (F-format string=w64:string)  [unwired: 2 in]
              n294 = Set File Position(refnum=w118, from (0:start)=enum16{"start", "end", "current"}."end" ("自（0:起始）"), error in=w119) -> (refnum out=w113:refnum<file>, error out=w112:errorcluster)  [unwired: 1 in]
              n295 = Concatenate Strings(w82, w99, w74, w89, w74, w85, w74, w97, w74, w96, w74, w95, w74, w94, w74, w88, w74, w66, w74, w65, w74, w64, w74, w63, w74, w62, w74, w61, "\r\n") -> (w83:string)
              n296 = Write to Text File(file (use dialog)=w113, text=w83, error in=w112) -> (refnum out=w105:refnum<file>, error out=w104:errorcluster)  [unwired: 1 in, 1 out]
            }
          }
        }
        n297 = VISA Close(VISA resource name=w8, error in (no error)=w7) -> ()  [unwired: 1 out]
        n298 = Close File(refnum=w4, error in=w3) -> ()  [unwired: 2 out]
        n299 = Close File(refnum=w6, error in=w5) -> ()  [unwired: 2 out]
      }
    }
  }
